vi "calibrateRfFreq.vi"(8 "error in (no error)":errorcluster, 9 "amplitude":string, 10 "channel_name":string, 11 "ChannelArray in":refnum<class "ChannelArray.lvclass">) -> (0 "error out":errorcluster, 2 "frequency":dbl, 3 "ChannelArray out":refnum<class "ChannelArray.lvclass">)   [LabVIEW 2009, in "Tools.lvlib" / "DatabaseHelpers.lvlib" / "ChannelArray.lvclass"]
uses:
  ChannelArray.lvclass
  Channel/RfOutputChannel/RfOutputChannel.lvclass
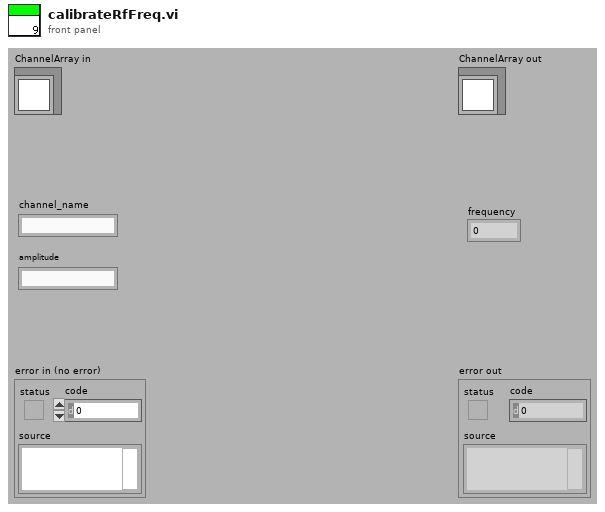
[diagram p1: front panel]
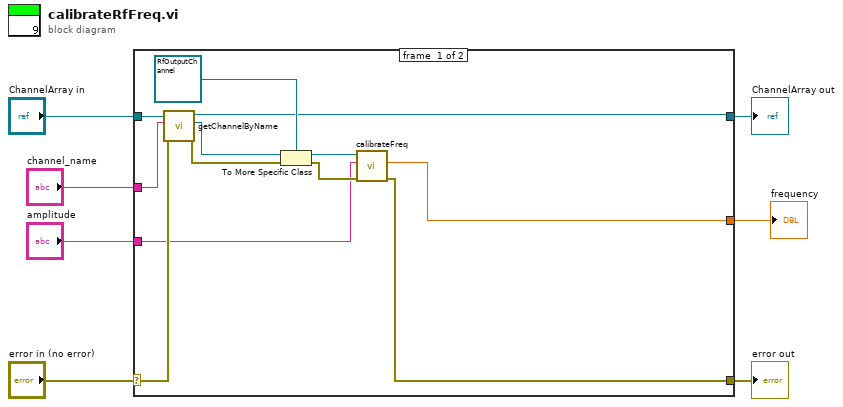
[diagram p0: block diagram]
diagram:
  n1 = case shown="No Error" "error in (no error)" {
    selector: "error in (no error)" -> [w17 w21]
    tunnel: [w8 w21] -> w6
    tunnel: [w13 w20] -> w4
    tunnel: "ChannelArray in" -> [w19 w20]
    tunnel: "channel_name" -> [w18 _]
    tunnel: "amplitude" -> [w10 _]
    tunnel: [w9 _] -> w1
    frame #0 {
      n2 = call-dynamic "getChannelByName.vi"("error in (no error)"=w17, "channel_name"=w18, "ChannelArray in"=w19) -> ("error out"=w14:errorcluster, "Channel"=w15:refnum<class "Channel.lvclass">, "ChannelArray out"=w13:refnum<class "ChannelArray.lvclass">)  [unwired: 5 in, 1 out]
      n3 = To More Specific Class(target class=refnum<class "RfOutputChannel.lvclass"> refnum ("RfOutputChannel in"), reference=w15, error in=w14) -> (specific class reference=w11:refnum<class "RfOutputChannel.lvclass">, error out=w12:errorcluster)
      n4 = call "calibrateFreq.vi"("error in (no error)"=w12, "value"=w10, "RfOutputChannel in"=w11) -> ("error out"=w8:errorcluster, "freq"=w9:dbl)  [unwired: 6 in, 1 out]
    }
    frame #1 {
    }
  }
  "error out" <- w6
  "ChannelArray out" <- w4
  "frequency" <- w1
